vi "Calculate Unscaled Response.vi"(0 "Neural Network In":refnum<class "Neural Network.lvclass">, 7 "Inputs":dbl[](array[numeric]), 11 "Error In":errorcluster) -> (4 "Neural Network Out":refnum<class "Neural Network.lvclass">, 8 "Unscaled Outputs":dbl[](array[numeric]), 15 "Error Out":errorcluster)   [LabVIEW 2015, in "Neural Network.lvclass"]
doc: "Calculate the output values of the network based on the input values. \n\nThis VI also uses the scaling information generated by the teaching algorithm to scale the inputs and outputs of the network. This means that you can work with any values as long as you have tought the network in that specific range."
uses:
  Neural Network.lvclass
  <vilib>/Analysis/NI_AALBase.lvlib
  <vilib>/Analysis/baseanly.llb/A x Vector.vi
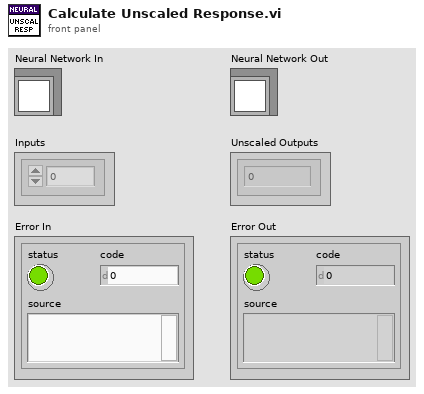
[diagram p1: front panel]
types:
  T1 = typedef "Neural Network.lvclass/2D Array.ctl" = cluster{"2D Array":sgl[][]}
  T2 = typedef "Neural Network.lvclass/Scaling Info.ctl" = cluster{"X Scaling Vector":dbl[], "Y Scaling Vector":dbl[]}
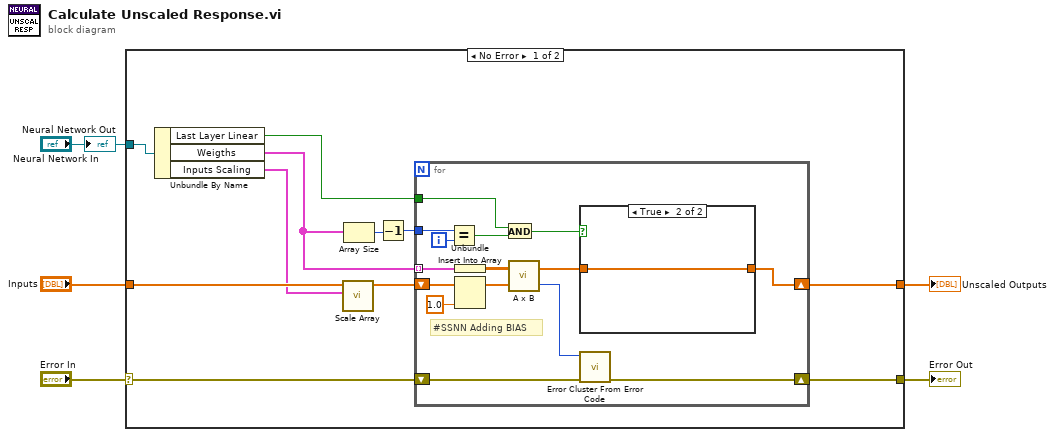
[diagram p0: block diagram]
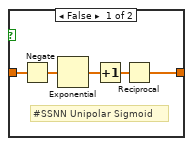
[diagram p2: hidden frame]
diagram:
  n1 = case shown="No Error" "Error In" {
    selector: "Error In" -> [w7 w38]
    tunnel: "Neural Network In" -> [w16 _]
    tunnel: "Inputs" -> [w13 _]
    tunnel: [w15 w38] -> w2
    tunnel: [w6 _] -> w1
    frame No Error {
      n2 = Unbundle By Name(w16) -> ("Last Layer Linear"=w14:bool, "Weigths"=w8:T1[], "Inputs Scaling"=w12:T2)
      n3 = call "Scale Array.vi"("Scaling Info"=w12, "Array to Scale"=w13) -> ("Scaled Array"=w9:dbl[])  [unwired: 9 in]
      n4 = Array Size(array=w8) -> (size(s)=w11:i32)
      n5 = Decrement(x=w11) -> (x-1=w10:i32)
      n6 = for {
        shift-right: [w29] -> w6
        shift-left: w9 -> [w28]
        tunnel: w8 -> [w31] mode=indexing
        tunnel: w10 -> [w25]
        shift-right: [w18] -> w15
        shift-left: w7 -> [w19]
        tunnel: w14 -> [w20]
        i -> [w23]
        # "#SSNN Adding BIAS"
        n7 = Equal?(x=w25, y=w23) -> (x = y?=w24:bool)
        n8 = Unbundle(w31) -> ("2D Array"=w30:sgl[][])
        n9 = Insert Into Array(array=w28, new element=1.0 ("new element/subarray")) -> (w27:dbl[])  [unwired: 1 in]
        n10 = And(x=w20, y=w24) -> (x .and. y?=w21:bool)
        n11 = call-poly <vilib>:"A x B.vi"("Vector"=w27, "A"=w30) -> ("error"=w22:i32, "A x Vector"=w26:dbl[])
        n12 = case shown="True" w21 {
          tunnel: [w33 w37] -> w29
          tunnel: w26 -> [w32 w37]
          frame False {
            # "#SSNN Unipolar Sigmoid"
            n13 = Negate(x=w32) -> (-x=w36:dbl[])
            n14 = Exponential(1:w36) -> (0:w35:dbl[])
            n15 = Increment(x=w35) -> (x+1=w34:dbl[])
            n16 = Reciprocal(x=w34) -> (1/x=w33:dbl[])
          }
          frame True {
          }
        }
        n17 = call <vilib>:"Error Cluster From Error Code.vi"("error in (no error)"=w19, "error code (0)"=w22) -> ("error out"=w18:errorcluster)  [unwired: 7 in]
      }
    }
    frame Error {
    }
  }
  "Error Out" <- w2
  "Unscaled Outputs" <- w1
  "Neural Network Out" <- "Neural Network In"
